vi "Create File Path.vi"(8 "error in":errorcluster, 11 "Report in":refnum<class "Report.lvclass">) -> (0 "error out":errorcluster, 3 "Report out":refnum<class "Report.lvclass">)   [LabVIEW 2023, in "Report.lvlib" / "Report.lvclass"]
uses:
  Report.lvclass
  Report.lvclass/Report.ctl
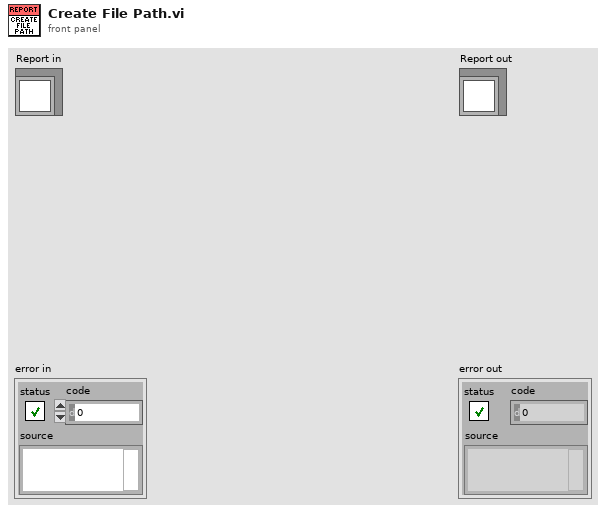
[diagram p1: front panel]
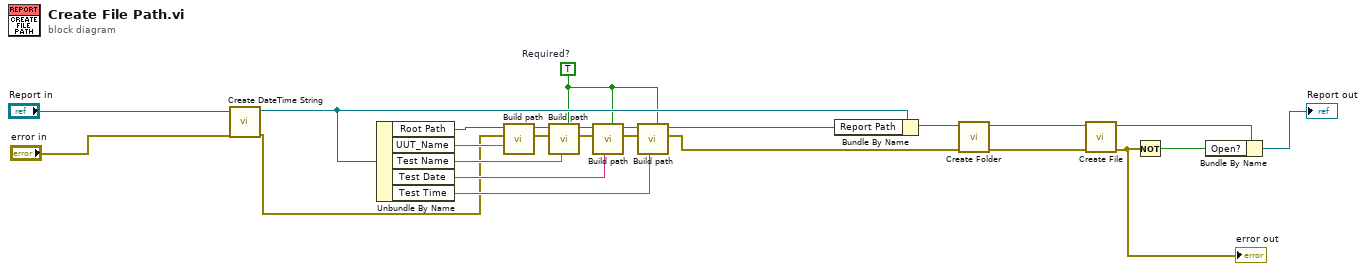
[diagram p0: block diagram]
diagram:
  w1 = TRUE  # Required?
  n1 = call "Create DateTime String.vi"("error in (no error)"="error in", "Report in"="Report in") -> ("error out"=w7:errorcluster, "Report out"=w8:refnum<class "Report.lvclass">)  [unwired: 8 in]
  n2 = Unbundle By Name(w8) -> ("Root Path"=w24:path, "UUT_Name"=w23:string, "Test Name"=w20:string, "Test Date"=w15:string, "Test Time"=w14:string)
  n3 = call "Build path.vi"("String"=w23, "error in"=w7, "Path"=w24) -> ("error out"=w21:errorcluster, "Path Out"=w22:path)  [unwired: 7 in]
  n4 = call "Build path.vi"("Required?"=w1, "String"=w20, "error in"=w21, "Path"=w22) -> ("error out"=w19:errorcluster, "Path Out"=w18:path)  [unwired: 6 in]
  n5 = call "Build path.vi"("Required?"=w1, "String"=w15, "error in"=w19, "Path"=w18) -> ("error out"=w17:errorcluster, "Path Out"=w16:path)  [unwired: 6 in]
  n6 = call "Build path.vi"("Required?"=w1, "String"=w14, "error in"=w17, "Path"=w16) -> ("error out"=w11:errorcluster, "Path Out"=w13:path)  [unwired: 6 in]
  n7 = Bundle By Name(cluster=w8, "Report Path"=w13) -> (w12:refnum<class "Report.lvclass">)
  n8 = call "Create Folder.vi"("error in"=w11, "Report in"=w12) -> ("error out"=w9:errorcluster, "Report out"=w10:refnum<class "Report.lvclass">)  [unwired: 8 in]
  n9 = call-dynamic "Create File.vi"("error in (no error)"=w9, "Report in"=w10) -> ("error out"=w3:errorcluster, "Report out"=w25:refnum<class "Report.lvclass">)  [unwired: 8 in]
  "error out" <- w3
  n10 = Not(x=w3) -> (.not. x?=w2:bool)
  n11 = Bundle By Name(cluster=w25, "Open?"=w2) -> (→"Report out":refnum<class "Report.lvclass">)
